vi "GetParam.vi"(8 "error in (no error)":errorcluster caption="entrée d'erreur (pas d'erreur)", 11 "Checkerboard.lvclass":refnum<class "Checkerboard.lvclass">) -> (0 "error out":errorcluster caption="sortie d'erreur", 2 "make_checkerboard":T1={"shape"={"n_rows"=300, "n_cols"=300}, "n_clusters"="5", "noise"=0.0, "minval"=10, "maxval"=100, "shuffle"=TRUE, "random_state"=-1, "Returns"="X"} {"shape"."n_cols" min=1; "shape"."n_rows" min=1; "random_state" min=-1}, 3 "Checkerboard.lvclass":refnum<class "Checkerboard.lvclass">)   [LabVIEW 2020, in "Checkerboard.lvclass"]
doc: "Get Parameters"
uses:
  Checkerboard.lvclass
  Checkerboard.lvclass/Checkerboard.ctl
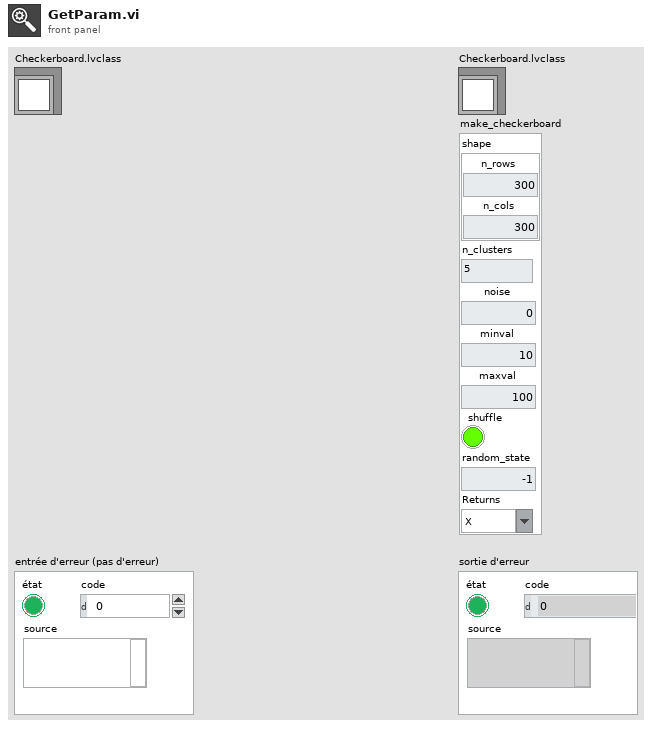
[diagram p1: front panel]
types:
  T1 = cluster{"shape":cluster{"n_rows":u32, "n_cols":u32}, "n_clusters":string, "noise":dbl, "minval":i32, "maxval":i32, "shuffle":bool, "random_state":i32, "Returns":string}
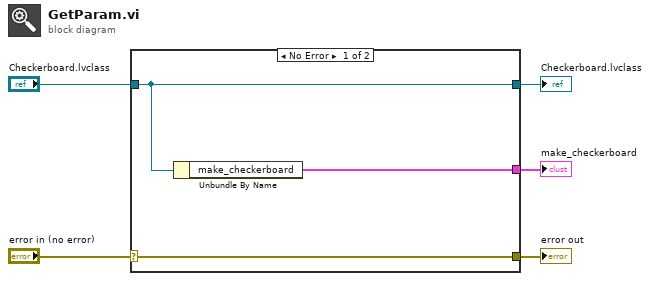
[diagram p0: block diagram]
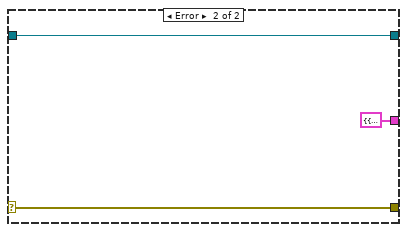
[diagram p2: hidden frame]
diagram:
  n1 = case shown="No Error" "error in (no error)" {
    selector: "error in (no error)" -> [w8 w10]
    tunnel: [w8 w10] -> w4
    tunnel: [w7 w11] -> w2
    tunnel: "Checkerboard.lvclass" -> [w7 w11]
    tunnel: [w6 T1 {"shape"={"n_rows"=0, "n_cols"=0}, "n_clusters"="", "noise"=0.0, "minval"=0, "maxval"=0, "shuffle"=FALSE, "random_state"=0, "Returns"=""} ("make_checkerboard")] -> w1
    frame No Error {
      n2 = Unbundle By Name(w7) -> ("make_checkerboard"=w6:T1)
    }
    frame Error {
    }
  }
  "error out" <- w4
  "Checkerboard.lvclass" <- w2
  "make_checkerboard" <- w1
